vi "Intake_set.vi"   [LabVIEW 2020]
uses:
  Globals/Intake_Motor_global.vi
  Intake_control_states.ctl
types:
  T1 = typedef "Intake_control_states.ctl" = enum16{"Manual_op", "No_Op"}
  T2 = typedef "Intake_cluster.ctl" = cluster{"control_states":T1, "Manual_control":dbl, "Trigger?":bool}
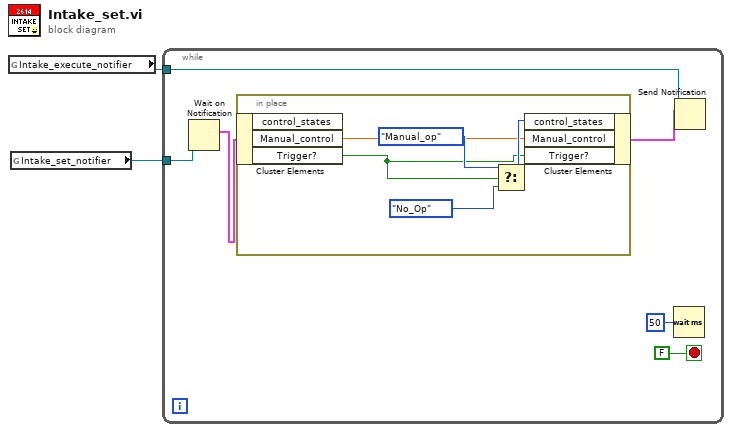
[diagram p0: block diagram]
diagram:
  n1 = global read "Intake_Motor_global.vi" "Intake_execute_notifier"() -> (w2:refnum<notifier>)
  n2 = global read "Intake_Motor_global.vi" "Intake_set_notifier"() -> (w1:refnum<notifier>)
  n3 = while {
    tunnel: w1 -> [w8]
    tunnel: w2 -> [w4]
    stop <- FALSE stop-if-true
    n4 = Wait on Notification(notifier=w8) -> (notification=w5:T2)  [unwired: 3 in, 3 out]
    n5 = in-place {
      n6 = in-place-cluster #1(w5) -> ("Manual_control"=w10:dbl, "Trigger?"=w9:bool)  [unwired: 1 out]
      n7 = Select(t=Intake_control_states."Manual_op" ("control_states"), s=w9, f=Intake_control_states."No_Op" ("control_states")) -> (s? t:f=w11:T1)
      n8 = in-place-cluster #1("control_states"=w11, "Manual_control"=w10, "Trigger?"=w9) -> (w3:T2)
    }
    n9 = Wait (ms)(milliseconds to wait=u32 50) -> ()  [unwired: 1 out]
    n10 = Send Notification(notification=w3, notifier=w4) -> ()  [unwired: 1 in, 2 out]
  }
